vi "CMI Sync V3 Set Channel 2 Mode.vi"(8 "error in":errorcluster, 10 "Channel 2 mode (DIV)":T1, 11 "session in":T2={"VISA"="", "baud rate [bd/s]"=115200, "source"=enum."Auto", "hv range"=enum."1kV", "fsrc is fixed"=FALSE, "fsrc [Hz]"=10000000.0, "freq integ [s]"=1.0, "freq filter"=5, "trig level"=enum."TTL 5V", "chn1 mode"=enum."Source divider", "chn1 level"=enum."Positive 5V", "chn2 mode"=enum."Source divider", "chn2 level"=enum."Positive 5V", "chn2 div"=1, "chn3 mode"=enum."Chn 1 Active", "chn3 level"=enum."Positive 5V", "chn1 div entry"=enum."Calculate nearest divisor from measured fx", "chn1 dev limit [%]"=1.0, "chn1 check dev"=FALSE} {"chn2 div" min=1 max=100000000 step=1; "fsrc [Hz]" format="%_8p"}) -> (0 "error out":errorcluster, 3 "session out":T2={"VISA"="", "baud rate [bd/s]"=115200, "source"=enum."Auto", "hv range"=enum."1kV", "fsrc is fixed"=FALSE, "fsrc [Hz]"=10000000.0, "freq integ [s]"=1.0, "freq filter"=5, "trig level"=enum."TTL 5V", "chn1 mode"=enum."Source divider", "chn1 level"=enum."Positive 5V", "chn2 mode"=enum."Source divider", "chn2 level"=enum."Positive 5V", "chn2 div"=1, "chn3 mode"=enum."Chn 1 Active", "chn3 level"=enum."Positive 5V", "chn1 div entry"=enum."Calculate nearest divisor from measured fx", "chn1 dev limit [%]"=1.0, "chn1 check dev"=FALSE} {"chn2 div" min=1 max=100000000 step=1; "fsrc [Hz]" format="%_8p"})   [LabVIEW 2020, in "AWG.lvlib" / "CMI Sync Unit V3.lvlib"]
doc: "Sets mode of channel 2."
uses:
  CMI Sync Unit V3.lvlib
  CMI Sync V3 session.ctl
  CMI Sync V3 Reference Clock Source.ctl
  CMI Sync V3 HV input Range.ctl
  CMI Sync V3 Trigger Input Level.ctl
  CMI Sync V3 Channel 1 Mode.ctl
  CMI Sync V3 Channel Output Levels.ctl
  CMI Sync V3 Channel 2 Mode.ctl
  CMI Sync V3 Channel 3 Mode.ctl
  CMI Sync V3 Channel 1 Divisor Entry Mode.ctl
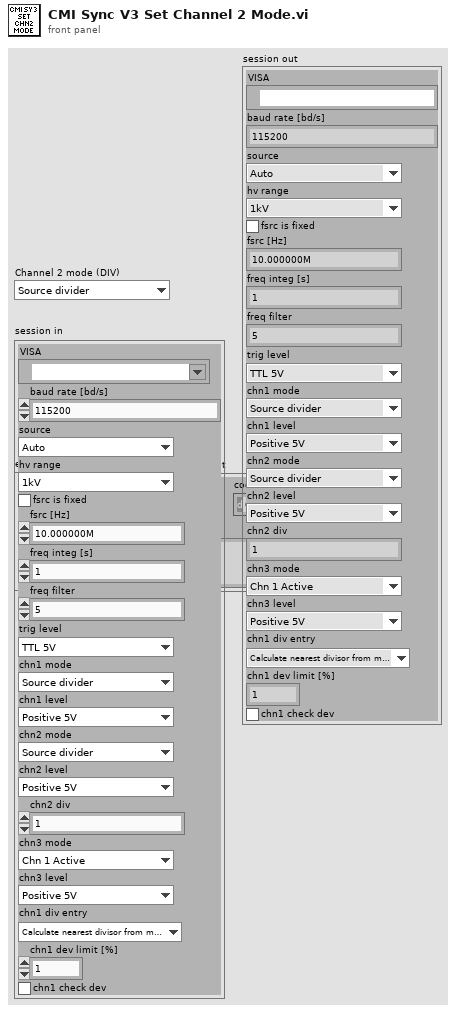
[diagram p1: front panel]
types:
  T1 = typedef "AWG.lvlib/CMI Sync Unit V3.lvlib/CMI Sync V3 Channel 2 Mode.ctl" = enum16{"Source divider", "Chn 1 divide"}
  T2 = typedef "AWG.lvlib/CMI Sync Unit V3.lvlib/CMI Sync V3 session.ctl" = cluster{"VISA":refnum<visa-resource-name>, "baud rate [bd/s]":i32, "source":T3, "hv range":T4, "fsrc is fixed":bool, "fsrc [Hz]":dbl, "freq integ [s]":dbl, "freq filter":i32, "trig level":T5, "chn1 mode":T6, "chn1 level":T7, "chn2 mode":T1, "chn2 level":T7, "chn2 div":i32, "chn3 mode":T8, "chn3 level":T7, "chn1 div entry":T9, "chn1 dev limit [%]":dbl, "chn1 check dev":bool}
  T3 = typedef "AWG.lvlib/CMI Sync Unit V3.lvlib/CMI Sync V3 Reference Clock Source.ctl" = enum16{"Auto", "Internal", "Logic", "Sine", "HV"}
  T4 = typedef "AWG.lvlib/CMI Sync Unit V3.lvlib/CMI Sync V3 HV input Range.ctl" = enum16{"10V", "60V", "250V", "1kV"}
  T5 = typedef "AWG.lvlib/CMI Sync Unit V3.lvlib/CMI Sync V3 Trigger Input Level.ctl" = enum16{"LVCMOS 3V3", "TTL 5V"}
  T6 = typedef "AWG.lvlib/CMI Sync Unit V3.lvlib/CMI Sync V3 Channel 1 Mode.ctl" = enum16{"Source divider", "DDS absolute", "DDS ratio", "DDS ratio M/N"}
  T7 = typedef "AWG.lvlib/CMI Sync Unit V3.lvlib/CMI Sync V3 Channel Output Levels.ctl" = enum16{"Positive 3V3", "Negative 3V3", "Positive 5V", "Negative 5V"}
  T8 = typedef "AWG.lvlib/CMI Sync Unit V3.lvlib/CMI Sync V3 Channel 3 Mode.ctl" = enum16{"Chn 1 Active", "Chn 2 Active", "Chn 1 Trigger", "Chn 2 Trigger", "Gate", "PPS", "10MHz"}
  T9 = typedef "AWG.lvlib/CMI Sync Unit V3.lvlib/CMI Sync V3 Channel 1 Divisor Entry Mode.ctl" = enum16{"Set divisor directly", "Calculate nearest divisor from measured fx"}
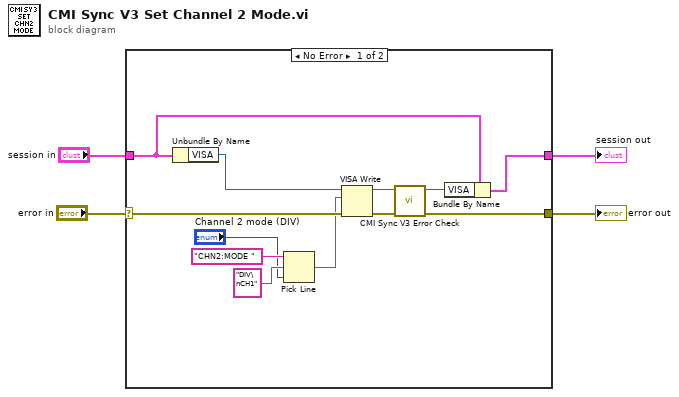
[diagram p0: block diagram]
diagram:
  n1 = case shown="No Error" "error in" {
    selector: "error in" -> [w8 w18]
    tunnel: "session in" -> [w16 w17]
    tunnel: [w15 w17] -> w1
    tunnel: [w10 w18] -> w2
    frame No Error {
      n2 = Unbundle By Name(w16) -> ("VISA"=w14:refnum<visa-resource-name>)
      n3 = Pick Line(string ("")="CHN2:MODE " ("format string"), multi-line string="DIV\nCH1", line index="Channel 2 mode (DIV)") -> (output string=w7:string)
      n4 = VISA Write(VISA resource name=w14, write buffer=w7, error in (no error)=w8) -> (VISA resource name out=w12:refnum<visa-resource-name>, error out=w13:errorcluster)  [unwired: 1 out]
      n5 = call "CMI Sync V3 Error Check.vi"("error in"=w13, "VISA in"=w12) -> ("error out"=w10:errorcluster, "VISA out"=w11:refnum<visa-resource-name>)  [unwired: 7 in, 1 out]
      n6 = Bundle By Name(cluster=w16, "VISA"=w11) -> (w15:T2)
    }
    frame Error {
    }
  }
  "error out" <- w2
  "session out" <- w1
